vi "real time object finder single cam 2 way v2.0 EJA 09 16 2016.vi"() -> ()   [LabVIEW 2011]
doc: "The Low-Level Grab VI acquires images continuously and displays the images in an image control using low-level acquisition VIs. A grab is appropriate for high-speed applications in which you need to process only one image at a time."
uses:
  <vilib>/userdefined/High Color/IMAQdx.ctl
  <vilib>/vision/driver/IMAQdx.llb/IMAQdx Buffer Number Mode.ctl
  <vilib>/Utility/file.llb/Write To Spreadsheet File (DBL).vi
  <vilib>/vision/driver/NI_Vision_Acquisition_Software.lvlib
  resource/objmgr/imaqdx.rc
  <vilib>/Analysis/NI_AALBase.lvlib
panel:
  in  "fish size":i32=10
  out "y position histogram":T1(graph)={"X Values"=[119.25, 147.75, 176.25, 204.75, 233.25, 261.75, 290.25, 318.75, 347.25, 375.75], "Histogram: h(x)"=[6, 5, 20, 28, 28, 24, 17, 8, 6, 9]}
  out "x position histogram":T1(graph)={"X Values"=[216.3, 244.9, 273.5, 302.1, 330.7, 359.3, 387.9, 416.5, 445.1, 473.7], "Histogram: h(x)"=[6, 14, 15, 13, 13, 22, 14, 24, 18, 12]}
  in  "histogram \nbins":i32=10
  in  "always save\non stop\nimaging":bool=TRUE
  in  "acquisition \ntime (s)":i32=5
  in  "save for a \ndesignated \nperiod":bool=TRUE
  out "trajectory":cluster{i32[], i32[]}(graph)={[360, 361, 361, 360, 360, 360, 354, 347, 332, 315, 297, 296, 303, 311, 322, 333, 345, 363, 373, 383, 390, 392, 393, 394, 394, 396, 402, 407, 408, 409, 411, 397, 379, 354, 331, 304, 283, 266, 249, 233, 219, 207, 202, 204, 213, 221, 238, 265, 294, 338, 340, 352, 353, 354, 355, 356, 360, 369, 391, 412, 414, 428, 442, 446, 459, 477, 481, 484, 488, 482, 475, 469, 467, 472, 475, 470, 463, 450, 441, 428, 417, 419, 426, 427, 424, 418, 404, 383, 359, 329, 306, 287, 274, 267, 259, 259, 257, 260, 270, 287, 300, 325, 336, 334, 332, 320, 306, 299, 291, 282, 274, 269, 264, 252, 252, 252, 249, 257, 253, 245, 249, 261, 277, 296, 322, 348, 369, 391, 410, 420, 421, 421, 421, 423, 428, 431, 435, 439, 446, 454, 459, 457, 454, 451, 449, 451, 445, 437, 424, 411, 395], [247, 247, 247, 250, 252, 257, 264, 274, 280, 284, 281, 275, 265, 247, 229, 211, 204, 198, 193, 192, 192, 192, 187, 173, 154, 140, 129, 109, 105, 108, 118, 129, 140, 152, 163, 173, 176, 180, 184, 190, 201, 223, 247, 271, 301, 324, 336, 335, 328, 315, 288, 270, 255, 255, 264, 274, 284, 288, 285, 265, 250, 239, 218, 206, 215, 214, 209, 211, 202, 192, 182, 179, 182, 199, 221, 250, 268, 270, 274, 283, 285, 290, 307, 355, 362, 353, 364, 373, 382, 387, 390, 390, 382, 368, 354, 340, 322, 308, 295, 284, 281, 278, 247, 227, 202, 178, 161, 165, 178, 197, 214, 229, 246, 254, 254, 255, 256, 245, 218, 201, 198, 199, 206, 222, 229, 230, 224, 215, 201, 189, 175, 168, 165, 170, 186, 204, 221, 232, 237, 239, 239, 237, 233, 229, 228, 242, 257, 276, 295, 308, 311]}
  in  "save\nlast\nimage":bool=TRUE
  in  "stop no save":bool
  out "date stub assigned":string="_2016Y_09M_15D_09h_48m_23s"
  in  "Acquire\ndata":bool
  in  "Experimental stub":string="danio01_test"
  out "Saving":bool
  in  "save data":bool
  in  "save path":path=path "E:/danio_tracking_2016/danio01_09_14_2016"
  in  "number\nformat (%.6f)":string="%.6f"
  in  "Marker\nText color":u32(colorbox)=16711680
  out "Multiplot":cluster{cluster{dbl, i32}[]}[](graph)=[{[{0.0, 360}, {0.033, 361}, {0.066, 361}, {0.1, 360}, {0.133, 360}, {0.166, 360}, {0.199, 354}, {0.233, 347}, {0.267, 332}, {0.3, 315}, {0.333, 297}, {0.366, 296}, {0.399, 303}, {0.433, 311}, {0.466, 322}, {0.499, 333}, {0.533, 345}, {0.566, 363}, {0.6, 373}, {0.633, 383}, {0.666, 390}, {0.7, 392}, {0.733, 393}, {0.767, 394}, {0.8, 394}, {0.833, 396}, {0.866, 402}, {0.899, 407}, {0.933, 408}, {0.967, 409}, {1.0, 411}, {1.033, 397}, {1.066, 379}, {1.1, 354}, {1.133, 331}, {1.166, 304}, {1.199, 283}, {1.232, 266}, {1.267, 249}, {1.3, 233}, {1.333, 219}, {1.366, 207}, {1.399, 202}, {1.433, 204}, {1.466, 213}, {1.499, 221}, {1.532, 238}, {1.566, 265}, {1.6, 294}, {1.633, 338}, {1.666, 340}, {1.699, 352}, {1.733, 353}, {1.767, 354}, {1.8, 355}, {1.833, 356}, {1.866, 360}, {1.899, 369}, {1.933, 391}, {1.967, 412}, {2.0, 414}, {2.033, 428}, {2.066, 442}, {2.1, 446}, {2.133, 459}, {2.167, 477}, {2.2, 481}, {2.233, 484}, {2.267, 488}, {2.3, 482}, {2.333, 475}, {2.366, 469}, {2.4, 467}, {2.434, 472}, {2.467, 475}, {2.5, 470}, {2.533, 463}, {2.566, 450}, {2.6, 441}, {2.634, 428}, {2.667, 417}, {2.7, 419}, {2.733, 426}, {2.767, 427}, {2.8, 424}, {2.833, 418}, {2.866, 404}, {2.899, 383}, {2.933, 359}, {2.967, 329}, {3.0, 306}, {3.033, 287}, {3.066, 274}, {3.1, 267}, {3.133, 259}, {3.166, 259}, {3.199, 257}, {3.232, 260}, {3.266, 270}, {3.3, 287}, {3.333, 300}, {3.366, 325}, {3.399, 336}, {3.433, 334}, {3.466, 332}, {3.5, 320}, {3.533, 306}, {3.566, 299}, {3.6, 291}, {3.633, 282}, {3.666, 274}, {3.699, 269}, {3.732, 264}, {3.766, 252}, {3.8, 252}, {3.833, 252}, {3.866, 249}, {3.899, 257}, {3.933, 253}, {3.966, 245}, {3.999, 249}, {4.033, 261}, {4.066, 277}, {4.1, 296}, {4.133, 322}, {4.166, 348}, {4.2, 369}, {4.233, 391}, {4.267, 410}, {4.3, 420}, {4.333, 421}, {4.366, 421}, {4.4, 421}, {4.434, 423}, {4.467, 428}, {4.5, 431}, {4.534, 435}, {4.566, 439}, {4.6, 446}, {4.634, 454}, {4.667, 459}, {4.7, 457}, {4.733, 454}, {4.777, 451}, {4.8, 449}, {4.835, 451}, {4.867, 445}, {4.9, 437}, {4.934, 424}, {4.967, 411}, {5.0, 395}]}, {[{0.0, 247}, {0.033, 247}, {0.066, 247}, {0.1, 250}, {0.133, 252}, {0.166, 257}, {0.199, 264}, {0.233, 274}, {0.267, 280}, {0.3, 284}, {0.333, 281}, {0.366, 275}, {0.399, 265}, {0.433, 247}, {0.466, 229}, {0.499, 211}, {0.533, 204}, {0.566, 198}, {0.6, 193}, {0.633, 192}, {0.666, 192}, {0.7, 192}, {0.733, 187}, {0.767, 173}, {0.8, 154}, {0.833, 140}, {0.866, 129}, {0.899, 109}, {0.933, 105}, {0.967, 108}, {1.0, 118}, {1.033, 129}, {1.066, 140}, {1.1, 152}, {1.133, 163}, {1.166, 173}, {1.199, 176}, {1.232, 180}, {1.267, 184}, {1.3, 190}, {1.333, 201}, {1.366, 223}, {1.399, 247}, {1.433, 271}, {1.466, 301}, {1.499, 324}, {1.532, 336}, {1.566, 335}, {1.6, 328}, {1.633, 315}, {1.666, 288}, {1.699, 270}, {1.733, 255}, {1.767, 255}, {1.8, 264}, {1.833, 274}, {1.866, 284}, {1.899, 288}, {1.933, 285}, {1.967, 265}, {2.0, 250}, {2.033, 239}, {2.066, 218}, {2.1, 206}, {2.133, 215}, {2.167, 214}, {2.2, 209}, {2.233, 211}, {2.267, 202}, {2.3, 192}, {2.333, 182}, {2.366, 179}, {2.4, 182}, {2.434, 199}, {2.467, 221}, {2.5, 250}, {2.533, 268}, {2.566, 270}, {2.6, 274}, {2.634, 283}, {2.667, 285}, {2.7, 290}, {2.733, 307}, {2.767, 355}, {2.8, 362}, {2.833, 353}, {2.866, 364}, {2.899, 373}, {2.933, 382}, {2.967, 387}, {3.0, 390}, {3.033, 390}, {3.066, 382}, {3.1, 368}, {3.133, 354}, {3.166, 340}, {3.199, 322}, {3.232, 308}, {3.266, 295}, {3.3, 284}, {3.333, 281}, {3.366, 278}, {3.399, 247}, {3.433, 227}, {3.466, 202}, {3.5, 178}, {3.533, 161}, {3.566, 165}, {3.6, 178}, {3.633, 197}, {3.666, 214}, {3.699, 229}, {3.732, 246}, {3.766, 254}, {3.8, 254}, {3.833, 255}, {3.866, 256}, {3.899, 245}, {3.933, 218}, {3.966, 201}, {3.999, 198}, {4.033, 199}, {4.066, 206}, {4.1, 222}, {4.133, 229}, {4.166, 230}, {4.2, 224}, {4.233, 215}, {4.267, 201}, {4.3, 189}, {4.333, 175}, {4.366, 168}, {4.4, 165}, {4.434, 170}, {4.467, 186}, {4.5, 204}, {4.534, 221}, {4.566, 232}, {4.6, 237}, {4.634, 239}, {4.667, 239}, {4.7, 237}, {4.733, 233}, {4.777, 229}, {4.8, 228}, {4.835, 242}, {4.867, 257}, {4.9, 276}, {4.934, 295}, {4.967, 308}, {5.0, 311}]}]
  out "FPS":i32=30
  out "time (s)":dbl[](array[numeric])=[0.0, 0.033, 0.066, 0.1, 0.133, 0.166, 0.199, 0.233, 0.267, 0.3, 0.333, 0.366, 0.399, 0.433, 0.466, 0.499, 0.533, 0.566, 0.6, 0.633, 0.666, 0.7, 0.733, 0.767, 0.8, 0.833, 0.866, 0.899, 0.933, 0.967, 1.0, 1.033, 1.066, 1.1, 1.133, 1.166, 1.199, 1.232, 1.267, 1.3, 1.333, 1.366, 1.399, 1.433, 1.466, 1.499, 1.532, 1.566, 1.6, 1.633, 1.666, 1.699, 1.733, 1.767, 1.8, 1.833, 1.866, 1.899, 1.933, 1.967, 2.0, 2.033, 2.066, 2.1, 2.133, 2.167, 2.2, 2.233, 2.267, 2.3, 2.333, 2.366, 2.4, 2.434, 2.467, 2.5, 2.533, 2.566, 2.6, 2.634, 2.667, 2.7, 2.733, 2.767, 2.8, 2.833, 2.866, 2.899, 2.933, 2.967, 3.0, 3.033, 3.066, 3.1, 3.133, 3.166, 3.199, 3.232, 3.266, 3.3, 3.333, 3.366, 3.399, 3.433, 3.466, 3.5, 3.533, 3.566, 3.6, 3.633, 3.666, 3.699, 3.732, 3.766, 3.8, 3.833, 3.866, 3.899, 3.933, 3.966, 3.999, 4.033, 4.066, 4.1, 4.133, 4.166, 4.2, 4.233, 4.267, 4.3, 4.333, 4.366, 4.4, 4.434, 4.467, 4.5, 4.534, 4.566, 4.6, 4.634, 4.667, 4.7, 4.733, 4.777, 4.8, 4.835, 4.867, 4.9, 4.934, 4.967, 5.0] format="%.3f"
  in  "Origin":cluster{"X":i32, "Y":i32}
  out "Y position vs time":cluster{dbl[], i32[]}(graph)={[0.0, 0.033, 0.066, 0.1, 0.133, 0.166, 0.199, 0.233, 0.267, 0.3, 0.333, 0.366, 0.399, 0.433, 0.466, 0.499, 0.533, 0.566, 0.6, 0.633, 0.666, 0.7, 0.733, 0.767, 0.8, 0.833, 0.866, 0.899, 0.933, 0.967, 1.0, 1.033, 1.066, 1.1, 1.133, 1.166, 1.199, 1.232, 1.267, 1.3, 1.333, 1.366, 1.399, 1.433, 1.466, 1.499, 1.532, 1.566, 1.6, 1.633, 1.666, 1.699, 1.733, 1.767, 1.8, 1.833, 1.866, 1.899, 1.933, 1.967, 2.0, 2.033, 2.066, 2.1, 2.133, 2.167, 2.2, 2.233, 2.267, 2.3, 2.333, 2.366, 2.4, 2.434, 2.467, 2.5, 2.533, 2.566, 2.6, 2.634, 2.667, 2.7, 2.733, 2.767, 2.8, 2.833, 2.866, 2.899, 2.933, 2.967, 3.0, 3.033, 3.066, 3.1, 3.133, 3.166, 3.199, 3.232, 3.266, 3.3, 3.333, 3.366, 3.399, 3.433, 3.466, 3.5, 3.533, 3.566, 3.6, 3.633, 3.666, 3.699, 3.732, 3.766, 3.8, 3.833, 3.866, 3.899, 3.933, 3.966, 3.999, 4.033, 4.066, 4.1, 4.133, 4.166, 4.2, 4.233, 4.267, 4.3, 4.333, 4.366, 4.4, 4.434, 4.467, 4.5, 4.534, 4.566, 4.6, 4.634, 4.667, 4.7, 4.733, 4.777, 4.8, 4.835, 4.867, 4.9, 4.934, 4.967, 5.0], [247, 247, 247, 250, 252, 257, 264, 274, 280, 284, 281, 275, 265, 247, 229, 211, 204, 198, 193, 192, 192, 192, 187, 173, 154, 140, 129, 109, 105, 108, 118, 129, 140, 152, 163, 173, 176, 180, 184, 190, 201, 223, 247, 271, 301, 324, 336, 335, 328, 315, 288, 270, 255, 255, 264, 274, 284, 288, 285, 265, 250, 239, 218, 206, 215, 214, 209, 211, 202, 192, 182, 179, 182, 199, 221, 250, 268, 270, 274, 283, 285, 290, 307, 355, 362, 353, 364, 373, 382, 387, 390, 390, 382, 368, 354, 340, 322, 308, 295, 284, 281, 278, 247, 227, 202, 178, 161, 165, 178, 197, 214, 229, 246, 254, 254, 255, 256, 245, 218, 201, 198, 199, 206, 222, 229, 230, 224, 215, 201, 189, 175, 168, 165, 170, 186, 204, 221, 232, 237, 239, 239, 237, 233, 229, 228, 242, 257, 276, 295, 308, 311]}
  out "X position vs time":cluster{dbl[], i32[]}(graph)={[0.0, 0.033, 0.066, 0.1, 0.133, 0.166, 0.199, 0.233, 0.267, 0.3, 0.333, 0.366, 0.399, 0.433, 0.466, 0.499, 0.533, 0.566, 0.6, 0.633, 0.666, 0.7, 0.733, 0.767, 0.8, 0.833, 0.866, 0.899, 0.933, 0.967, 1.0, 1.033, 1.066, 1.1, 1.133, 1.166, 1.199, 1.232, 1.267, 1.3, 1.333, 1.366, 1.399, 1.433, 1.466, 1.499, 1.532, 1.566, 1.6, 1.633, 1.666, 1.699, 1.733, 1.767, 1.8, 1.833, 1.866, 1.899, 1.933, 1.967, 2.0, 2.033, 2.066, 2.1, 2.133, 2.167, 2.2, 2.233, 2.267, 2.3, 2.333, 2.366, 2.4, 2.434, 2.467, 2.5, 2.533, 2.566, 2.6, 2.634, 2.667, 2.7, 2.733, 2.767, 2.8, 2.833, 2.866, 2.899, 2.933, 2.967, 3.0, 3.033, 3.066, 3.1, 3.133, 3.166, 3.199, 3.232, 3.266, 3.3, 3.333, 3.366, 3.399, 3.433, 3.466, 3.5, 3.533, 3.566, 3.6, 3.633, 3.666, 3.699, 3.732, 3.766, 3.8, 3.833, 3.866, 3.899, 3.933, 3.966, 3.999, 4.033, 4.066, 4.1, 4.133, 4.166, 4.2, 4.233, 4.267, 4.3, 4.333, 4.366, 4.4, 4.434, 4.467, 4.5, 4.534, 4.566, 4.6, 4.634, 4.667, 4.7, 4.733, 4.777, 4.8, 4.835, 4.867, 4.9, 4.934, 4.967, 5.0], [360, 361, 361, 360, 360, 360, 354, 347, 332, 315, 297, 296, 303, 311, 322, 333, 345, 363, 373, 383, 390, 392, 393, 394, 394, 396, 402, 407, 408, 409, 411, 397, 379, 354, 331, 304, 283, 266, 249, 233, 219, 207, 202, 204, 213, 221, 238, 265, 294, 338, 340, 352, 353, 354, 355, 356, 360, 369, 391, 412, 414, 428, 442, 446, 459, 477, 481, 484, 488, 482, 475, 469, 467, 472, 475, 470, 463, 450, 441, 428, 417, 419, 426, 427, 424, 418, 404, 383, 359, 329, 306, 287, 274, 267, 259, 259, 257, 260, 270, 287, 300, 325, 336, 334, 332, 320, 306, 299, 291, 282, 274, 269, 264, 252, 252, 252, 249, 257, 253, 245, 249, 261, 277, 296, 322, 348, 369, 391, 410, 420, 421, 421, 421, 423, 428, 431, 435, 439, 446, 454, 459, 457, 454, 451, 449, 451, 445, 437, 424, 411, 395]}
  in  "Pixel intensity\nthreshold":i32=90
  in  "Row min":i32=10
  in  "Row max":i32=470
  in  "Column min":i32=10
  in  "Column max":i32=630
  out "X positions\ncamera 1\n(image \ncoordinates)":i32[](array[numeric])=[360, 361, 361, 360, 360, 360, 354, 347, 332, 315, 297, 296, 303, 311, 322, 333, 345, 363, 373, 383, 390, 392, 393, 394, 394, 396, 402, 407, 408, 409, 411, 397, 379, 354, 331, 304, 283, 266, 249, 233, 219, 207, 202, 204, 213, 221, 238, 265, 294, 338, 340, 352, 353, 354, 355, 356, 360, 369, 391, 412, 414, 428, 442, 446, 459, 477, 481, 484, 488, 482, 475, 469, 467, 472, 475, 470, 463, 450, 441, 428, 417, 419, 426, 427, 424, 418, 404, 383, 359, 329, 306, 287, 274, 267, 259, 259, 257, 260, 270, 287, 300, 325, 336, 334, 332, 320, 306, 299, 291, 282, 274, 269, 264, 252, 252, 252, 249, 257, 253, 245, 249, 261, 277, 296, 322, 348, 369, 391, 410, 420, 421, 421, 421, 423, 428, 431, 435, 439, 446, 454, 459, 457, 454, 451, 449, 451, 445, 437, 424, 411, 395]
  out "Y positions camera 1 \n(image \ncoordinates)":i32[](array[numeric])=[247, 247, 247, 250, 252, 257, 264, 274, 280, 284, 281, 275, 265, 247, 229, 211, 204, 198, 193, 192, 192, 192, 187, 173, 154, 140, 129, 109, 105, 108, 118, 129, 140, 152, 163, 173, 176, 180, 184, 190, 201, 223, 247, 271, 301, 324, 336, 335, 328, 315, 288, 270, 255, 255, 264, 274, 284, 288, 285, 265, 250, 239, 218, 206, 215, 214, 209, 211, 202, 192, 182, 179, 182, 199, 221, 250, 268, 270, 274, 283, 285, 290, 307, 355, 362, 353, 364, 373, 382, 387, 390, 390, 382, 368, 354, 340, 322, 308, 295, 284, 281, 278, 247, 227, 202, 178, 161, 165, 178, 197, 214, 229, 246, 254, 254, 255, 256, 245, 218, 201, 198, 199, 206, 222, 229, 230, 224, 215, 201, 189, 175, 168, 165, 170, 186, 204, 221, 232, 237, 239, 239, 237, 233, 229, 228, 242, 257, 276, 295, 308, 311]
  out "LIVE":bool
  in  "stop":bool
  out "Camera backlog":i32(slide)=-1 scale=0.0..50.0
  in  "IMAQdx Device Camera":T2="cam2"
  in  "Buffers Camera 1":u32=50
  out "Image":T3(plugin-control)
  # "PROGRAM INFO\n\nThis program finds the\nfirst pixel below the \nuser threshold in\nthe user specified\nROI below"
  # "Camera search ROI"
  # "Data acquisition \nsettings"
  # "issues\n\nHow do we know if frames \nare dropped?\n\nProbably will need to save data\nin sections to an open file\n\nCould have a sliding ROI based\non previous trailing edge position\n\nCould process each data chunk\nseparately to avoid frame dropping\nissues.  I.e. if you write every 1000\npoints, then in post processing only\nprocess 1000 at a time."
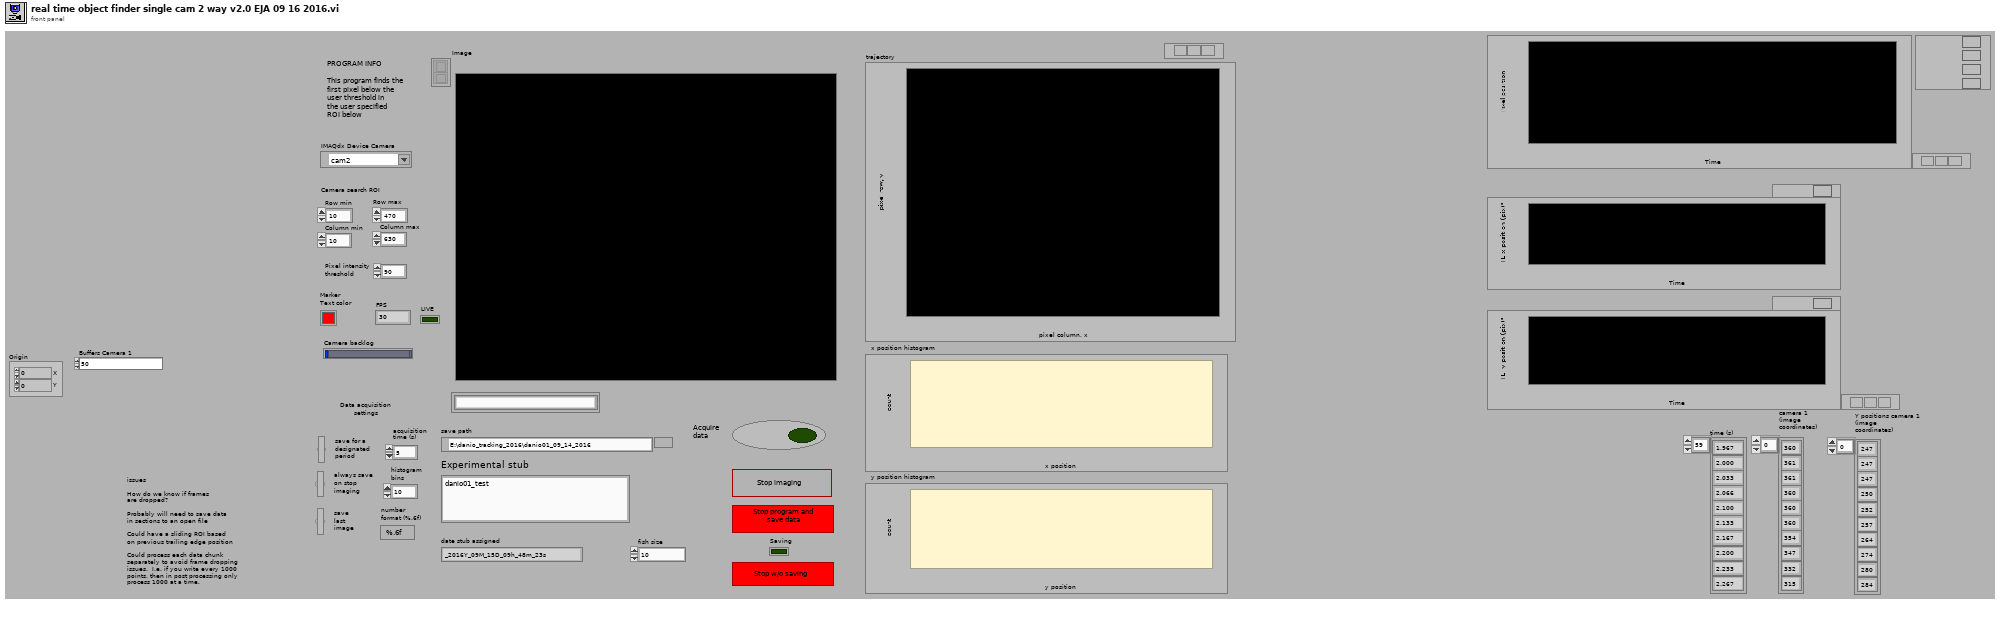
[diagram p1: front panel]
types:
  T1 = cluster{"X Values":dbl[], "Histogram: h(x)":i32[]}
  T2 = typedef "IMAQdx.ctl" = refnum<k21>
  T3 = typedef "IMAQ Image.ctl" = refnum<image>
  T4 = typedef "NI_Vision_Acquisition_Software.lvlib/IMAQdx Buffer Number Mode.ctl" = enum32{"Next", "Last", "Buffer Number"}
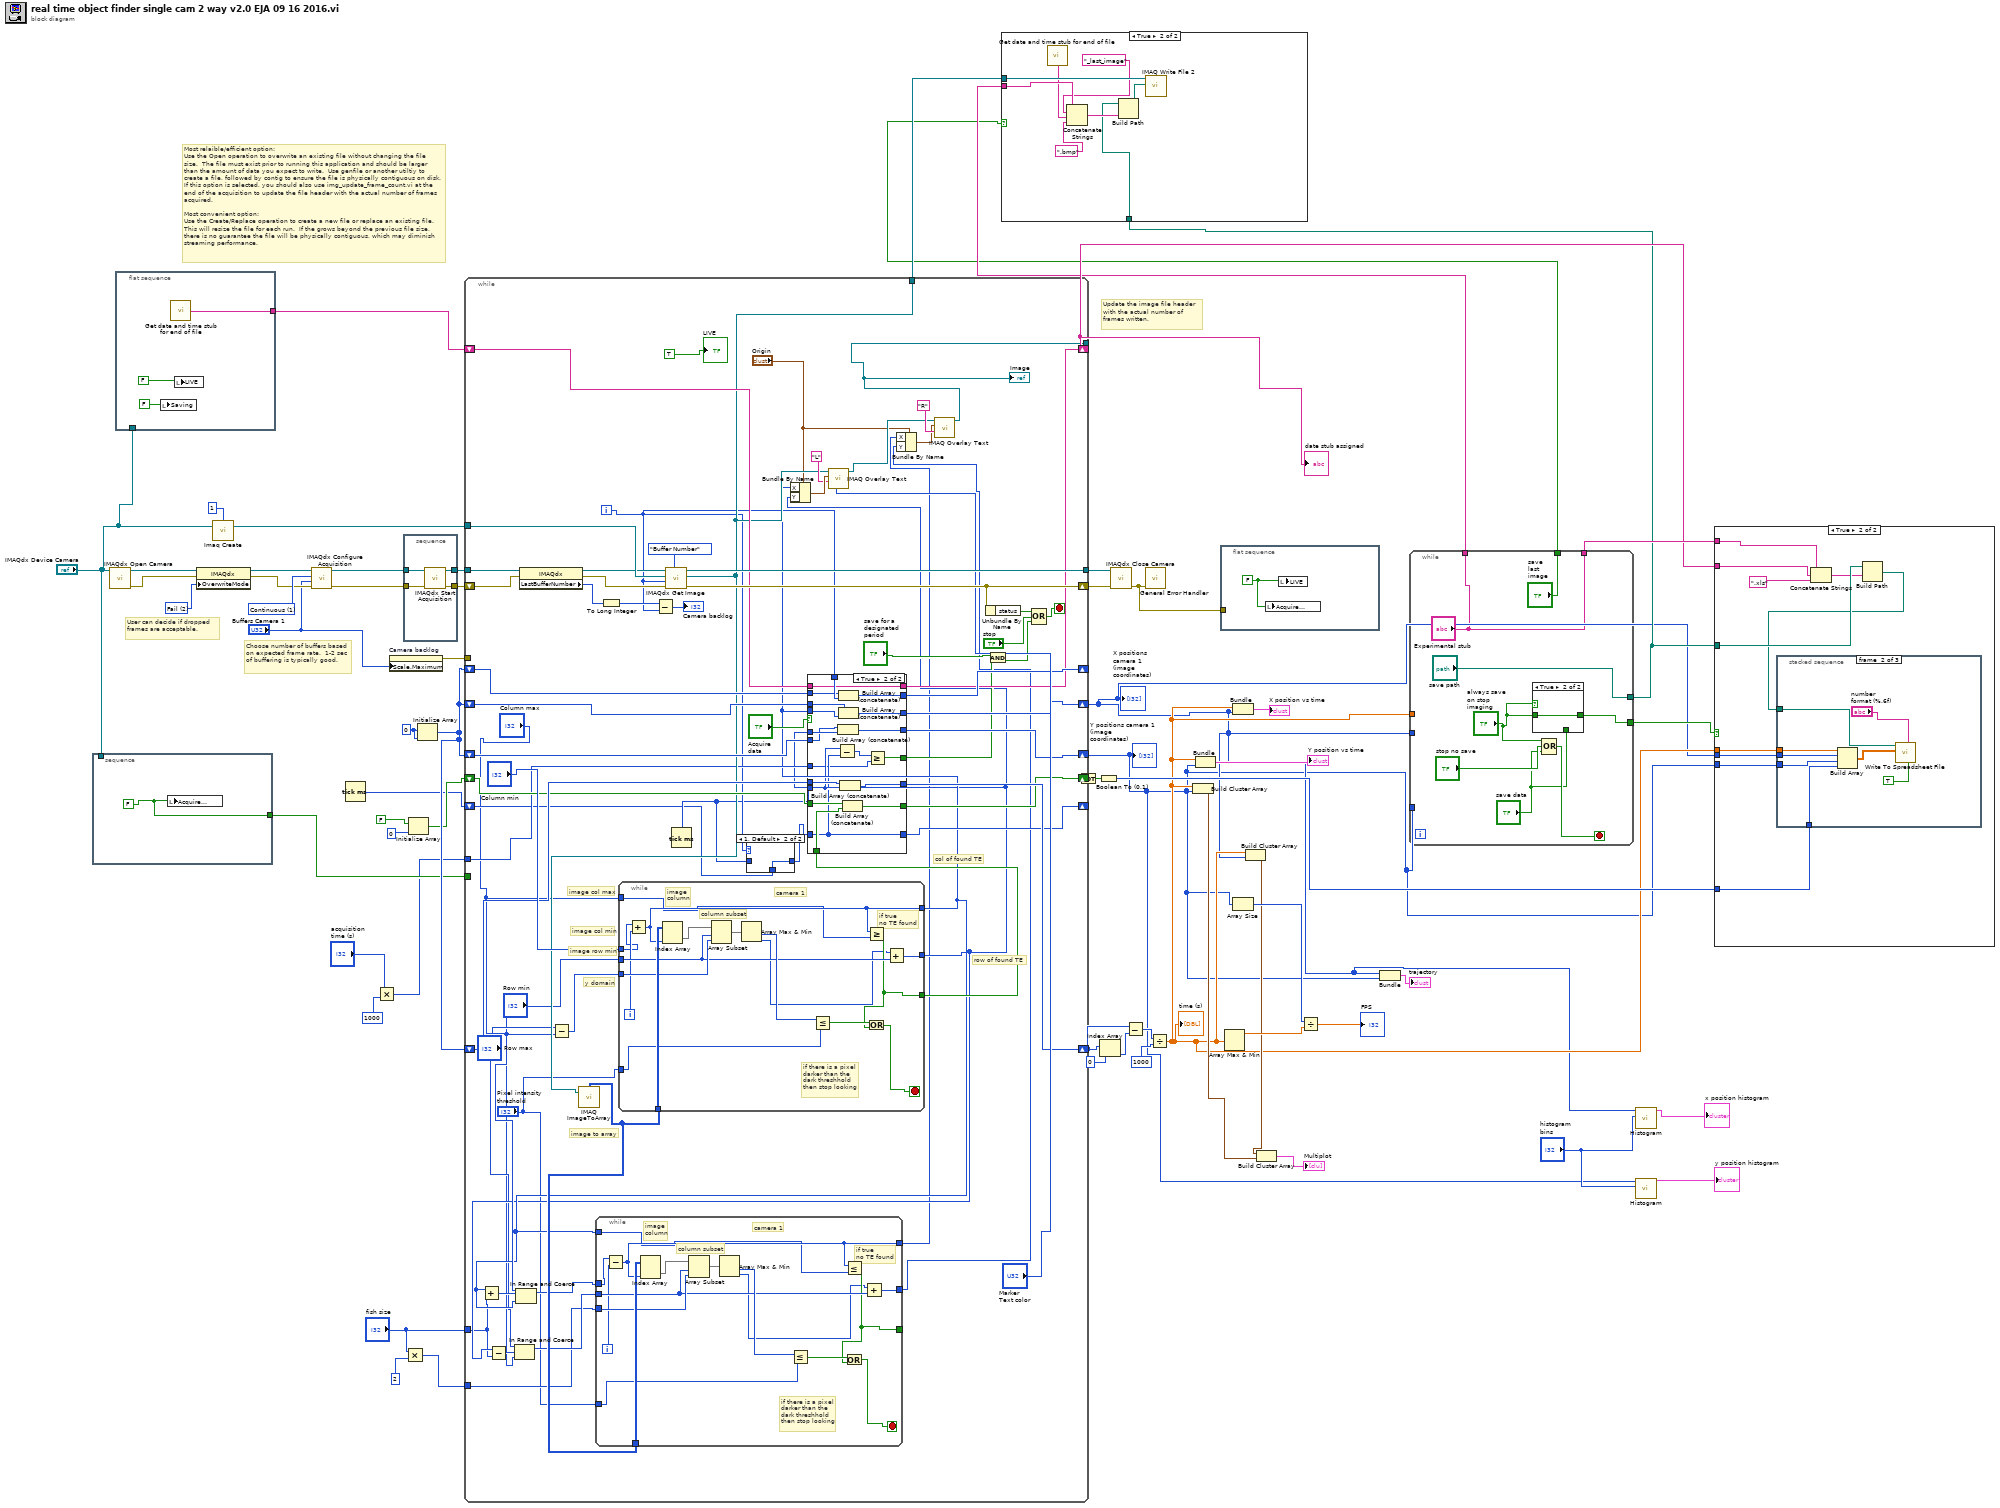
[diagram p0: block diagram]
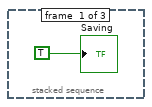
[diagram p4: hidden frame]
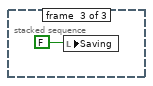
[diagram p5: hidden frame]
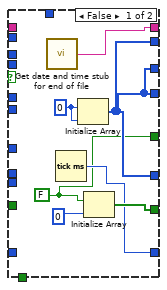
[diagram p8: hidden frame]
diagram:
  w31 = 0
  w55 = u32 2 items=["Get Oldest"=0, "Fail"=2, "Get Newest"=3] ("OverwriteMode")
  w61 = u32 1 items=["One Shot", "Continuous"] ("Continuous ?")
  # "Update the image file header with the actual number of frames written."
  # "Choose number of buffers based on expected frame rate.  1-2 sec of buffering is typically good."
  # "User can decide if dropped frames are acceptable."
  # "Most relaible/efficient option:\nUse the Open operation to overwrite an existing file without changing the file size.  The file must exist prior to running this application and should be larger than the amount of data you expect to write.  Use genfile or another utiltiy to create a file, followed by contig to ensure the file is physically contiguous on disk.  If this option is selected, you should also use img_update_frame_count.vi at the end of the acquisition to update the file header with the actual number of frames acquired. \n\nMost convenient option:\nUse the Create/Replace operation to create a new file or replace an existing file. This will resize the file for each run.  If the grows beyond the previous file size, there is no guarantee the file will be physically contiguous, which may diminish streaming performance."
  n1 = stacked-sequence {
    tunnel: "IMAQdx Device Camera" -> [_]
    tunnel: [w63] -> w15
    frame #0 {
      w63 = FALSE
      n2 = local write "Acquire\ndata"(w63) -> ()
    }
  }
  n3 = call <vilib>:"IMAQdx Open Camera.vi"("Session In"="IMAQdx Device Camera") -> ("error out"=w51:errorcluster, "Session Out"=w50:T2)  [unwired: 2 in, 7 out]
  n4 = flat-sequence {
    tunnel: "IMAQdx Device Camera" -> [_]
    tunnel: [w64] -> w30
    frame #0 {
      n5 = local write "Saving"(FALSE) -> ()
      n6 = call <userlib>:"Get date and time stub for end of file.vi"() -> ("date and time stub"=w64:string)
      n7 = local write "LIVE"(FALSE) -> ()
    }
  }
  n8 = property class="IMAQdx"(reference=w50, error in=w51, "OverwriteMode"=w55) -> (reference out=w53:T2, error out=w52:errorcluster)
  n9 = call "Imaq Create"("Border Size"=1, "Image Name"="IMAQdx Device Camera") -> ("New Image"=w62:T3)  [unwired: 2 in, 2 out]
  n10 = call <vilib>:"IMAQdx Configure Acquisition.vi"("error in"=w52, "Number of Buffers"="Buffers Camera 1", "Continuous?"=w61, "Session In"=w53) -> ("error out"=w47:errorcluster, "Session Out"=w54:T2)  [unwired: 6 out]
  n11 = Tick Count (ms)() -> (millisecond timer value=w9:u32)
  n12 = Multiply(x="acquisition \ntime (s)", y=1000) -> (x*y=w10:i32)
  n13 = property on="Camera backlog" class="Slide (strict)"("Scale.Maximum"="Buffers Camera 1") -> (error out=w49:errorcluster)  [unwired: 2 in, 1 out]
  n14 = stacked-sequence {
    tunnel: [w70] -> w60
    tunnel: [w69] -> w59
    tunnel: w54 -> [w68]
    tunnel: w47 -> [w67]
    frame #0 {
      n15 = call <vilib>:"IMAQdx Start Acquisition.vi"("error in"=w67, "Session In"=w68) -> ("error out"=w70:errorcluster, "Session Out"=w69:T2)  [unwired: 8 out]
    }
  }
  n16 = Multiply(x="fish size", y=2) -> (x*y=w1:i32)
  n17 = Initialize Array(FALSE, 0) -> (w22:bool[])
  n18 = Initialize Array(w31, w31) -> (w28:i32[])
  n19 = while {
    tunnel: [w129] -> w57
    tunnel: w59 -> [w132]
    tunnel: w62 -> [w130]
    tunnel: [w72] -> _
    shift-right: [w128] -> w56
    shift-left: w60 -> [w131]
    tunnel: w49 -> [_]
    shift-right: [w112] -> _
    shift-left: w28 -> [w113]
    shift-right: [w111] -> w8
    shift-left: w28 -> [w110]
    shift-right: [w109] -> w4
    shift-left: w28 -> [w108]
    shift-right: [w107] -> w41
    shift-left: w28 -> [w106]
    shift-right: [w104] -> w29
    shift-left: w30 -> [w105]
    shift-right: [w102] -> w27
    shift-left: w22 -> [w103]
    tunnel: [w100] -> w20
    tunnel: w15 -> [_]
    shift-right: [w99] -> _
    shift-left: w9 -> [w91]
    tunnel: w10 -> [w98]
    tunnel: "fish size" -> [w84]
    tunnel: w1 -> [w79]
    i -> [w94]
    stop <- w134 stop-if-true
    # "image col min"
    # "image col max"
    # "image row min"
    # "row of found TE"
    # "col of found TE"
    # "y domain"
    # "image to array"
    n20 = property class="IMAQdx"(reference=w132, error in=w131) -> (reference out=w125:T2, error out=w126:errorcluster, "LastBufferNumber"=w122:u32)
    n21 = Subtract(x="Row max", y="Row min") -> (x-y=w116:i32)
    n22 = To Long Integer(number=w122) -> (32bit integer=w121:i32)
    n23 = Subtract(x=w121, y=w94) -> (x-y=→"Camera backlog":i32)
    n24 = call <vilib>:"IMAQdx Get Image.vi"("Buffer Number Mode (Next)"=IMAQdx_Buffer_Number_Mode."Buffer Number", "error in"=w126, "Buffer Number In"=w94, "Image In"=w130, "Session In"=w125) -> ("error out"=w128:errorcluster, "Image Out"=w100:T3, "Session Out"=w129:T2)  [unwired: 1 in, 3 out]
    n25 = call "IMAQ ImageToArray"("Image"=w100) -> ("Image Pixels (U8)"=w90:u8[][])  [unwired: 2 in, 5 out]
    n26 = while {
      tunnel: "Row min" -> [w189]
      tunnel: [w188] -> w86
      tunnel: [w190] -> w85
      tunnel: w116 -> [w192]
      tunnel: w90 -> [w194]
      tunnel: "Column max" -> [w180]
      tunnel: "Column min" -> [w181]
      tunnel: [w185] -> w101
      tunnel: "Pixel intensity\nthreshold" -> [w183]
      i -> [w182]
      stop <- w186 stop-if-true
      # "if true\nno TE found"
      # "camera 1"
      # "if there is a pixel\ndarker than the\ndark threshhold\nthen stop looking"
      # "column subset"
      # "image\ncolumn"
      n27 = Add(x=w181, y=w182) -> (x+y=w188:i32)
      n28 = Index Array(array=w194, index (col)=w188) -> (element=w193:u8[])  [unwired: 1 in]
      n29 = Array Subset(array=w193, index=w189, length=w192) -> (w191:u8[])
      n30 = Array Max & Min(array=w191) -> (min value=w195:u8, min index (indices)=w184:i32)  [unwired: 2 out]
      n31 = Less Or Equal?(x=w195, y=w183) -> (x <= y?=w187:bool)
      n32 = Greater Or Equal?(x=w188, y=w180) -> (x >= y?=w185:bool)
      n33 = Or(x=w187, y=w185) -> (x .or. y?=w186:bool)
      n34 = Add(x=w184, y=w189) -> (x+y=w190:i32)
    }
    n35 = Add(x=w86, y=w84) -> (x+y=w89:i32)
    n36 = Subtract(x=w85, y=w84) -> (x-y=w83:i32)
    n37 = In Range and Coerce(upper limit="Row max", x=w83, lower limit="Row min") -> (coerced(x)=w80:i32)  [unwired: 1 out]
    n38 = In Range and Coerce(upper limit="Column max", x=w89, lower limit=w86) -> (coerced(x)=w87:i32)  [unwired: 1 out]
    n39 = while {
      tunnel: w80 -> [w144]
      tunnel: [w143] -> w74
      tunnel: [w145] -> w75
      tunnel: w79 -> [w147]
      tunnel: w90 -> [w149]
      tunnel: w86 -> [w135]
      tunnel: w87 -> [w136]
      tunnel: [w140] -> _
      tunnel: "Pixel intensity\nthreshold" -> [w138]
      i -> [w137]
      stop <- w141 stop-if-true
      # "if true\nno TE found"
      # "camera 1"
      # "if there is a pixel\ndarker than the\ndark threshhold\nthen stop looking"
      # "column subset"
      # "image\ncolumn"
      n40 = Subtract(x=w136, y=w137) -> (x-y=w143:i32)
      n41 = Index Array(array=w149, index (col)=w143) -> (element=w148:u8[])  [unwired: 1 in]
      n42 = Array Subset(array=w148, index=w144, length=w147) -> (w146:u8[])
      n43 = Array Max & Min(array=w146) -> (min value=w150:u8, min index (indices)=w139:i32)  [unwired: 2 out]
      n44 = Less Or Equal?(x=w150, y=w138) -> (x <= y?=w142:bool)
      n45 = Less Or Equal?(x=w143, y=w135) -> (x <= y?=w140:bool)
      n46 = Or(x=w142, y=w140) -> (x .or. y?=w141:bool)
      n47 = Add(x=w139, y=w144) -> (x+y=w145:i32)
    }
    n48 = Tick Count (ms)() -> (millisecond timer value=w93:u32)
    n49 = case shown="1, Default" w94 {
      tunnel: w93 -> [w151 _]
      tunnel: [w151 w152] -> w92
      tunnel: w91 -> [_ w152]
      frame 0 {
      }
      frame 1, Default {
      }
    }
    n50 = Bundle By Name(cluster="Origin", "X"=w86, "Y"=w85) -> (w119:cluster{"X":i32, "Y":i32})
    n51 = case shown="True" "Acquire\ndata" {
      tunnel: w94 -> [_ w179]
      tunnel: w113 -> [_ w178]
      tunnel: [w157 w177] -> w112
      tunnel: w86 -> [_ w175]
      tunnel: [w157 w176] -> w111
      tunnel: w110 -> [_ w174]
      tunnel: w85 -> [_ w173]
      tunnel: [w157 w172] -> w109
      tunnel: w108 -> [_ w171]
      tunnel: w93 -> [_ w163]
      tunnel: [w157 w170] -> w107
      tunnel: w106 -> [_ w169]
      tunnel: [w158 w168] -> w104
      tunnel: w105 -> [_ w168]
      tunnel: w103 -> [_ w167]
      tunnel: w101 -> [_ w166]
      tunnel: [w155 w165] -> w102
      tunnel: w92 -> [_ w162]
      tunnel: [w154 w162] -> w99
      tunnel: w98 -> [_ w161]
      tunnel: [w153 w160] -> w97
      frame False {
        w153 = FALSE
        w159 = 0
        n52 = call <userlib>:"Get date and time stub for end of file.vi"() -> ("date and time stub"=w158:string)
        n53 = Tick Count (ms)() -> (millisecond timer value=w154:u32)
        n54 = Initialize Array(w159, w159) -> (w157:i32[])
        n55 = Initialize Array(w153, 0) -> (w155:bool[])
      }
      frame True {
        n56 = Subtract(x=w163, y=w162) -> (x-y=w164:u32)
        n57 = Build Array (concatenate)(w171, w173) -> (w172:i32[])
        n58 = Build Array (concatenate)(w178, w179) -> (w177:i32[])
        n59 = Build Array (concatenate)(w174, w175) -> (w176:i32[])
        n60 = Build Array (concatenate)(w169, w163) -> (w170:u32[])
        n61 = Build Array (concatenate)(w167, w166) -> (w165:bool[])
        n62 = Greater Or Equal?(x=w164, y=w161) -> (x >= y?=w160:bool)
      }
    }
    n63 = call "IMAQ Overlay Text"("Text Color (black)"="Marker\nText color", "String"="L", "Origin"=w119, "Image"=w100) -> ("Image Out"=w73:T3)  [unwired: 4 in, 3 out]
    n64 = Bundle By Name(cluster="Origin", "X"=w74, "Y"=w75) -> (w76:cluster{"X":i32, "Y":i32})
    n65 = call "IMAQ Overlay Text"("String"="R", "Origin"=w76, "Image"=w73) -> ("Image Out"=w72:T3)  [unwired: 5 in, 3 out]
    "Image" <- w72
    n66 = Unbundle By Name(w128) -> ("status"=w133:bool)
    n67 = And(x="save for a \ndesignated \nperiod", y=w97) -> (x .and. y?=w96:bool)
    n68 = Compound Arithmetic op=OR(w133, "stop", w96) -> (w134:bool)
    "LIVE" <- TRUE
  }
  "X positions\ncamera 1\n(image \ncoordinates)" <- w8
  "Y positions camera 1 \n(image \ncoordinates)" <- w4
  "date stub assigned" <- w29
  n69 = Not(x=w27) -> (.not. x?=w24:bool[])
  n70 = Boolean To (0,1)(Boolean=w24) -> (0, 1=w23:i16[])
  n71 = Index Array(array=w41, index=0) -> (element=w42:u32)
  n72 = call <vilib>:"IMAQdx Close Camera.vi"("error in"=w56, "Session In"=w57) -> ("error out"=w46:errorcluster)  [unwired: 9 out]
  n73 = Subtract(x=w41, y=w42) -> (x-y=w36:u32[])
  n74 = call <vilib>:"General Error Handler.vi"("error in (no error)"=w46) -> ()  [unwired: 1 in, 14 out]
  n75 = Divide(x=w36, y=1000) -> (x/y=w14:dbl[])
  "time (s)" <- w14
  n76 = Build Cluster Array(w14, w4) -> (w33:cluster{dbl, i32}[])
  n77 = Bundle(w14, w4) -> (→"Y position vs time":cluster{dbl[], i32[]})  [unwired: 1 out]
  n78 = flat-sequence {
    tunnel: w46 -> [_]
    frame #0 {
      w196 = FALSE
      n79 = local write "Acquire\ndata"(w196) -> ()
      n80 = local write "LIVE"(w196) -> ()
    }
  }
  n81 = Array Max & Min(array=w14) -> (max value=w40:dbl)  [unwired: 3 out]
  n82 = Bundle(w14, w8) -> (→"X position vs time":cluster{dbl[], i32[]})  [unwired: 1 out]
  n83 = Array Size(array=w4) -> (size(s)=w39:i32)
  n84 = Build Cluster Array(w14, w8) -> (w34:cluster{dbl, i32}[])
  n85 = Build Cluster Array(w34, w33) -> (→"Multiplot":cluster{cluster{dbl, i32}[]}[])
  n86 = Divide(x=w39, y=w40) -> (x/y=→"FPS":dbl)
  n87 = Bundle(w8, w4) -> (→"trajectory":cluster{i32[], i32[]})  [unwired: 1 out]
  n88 = while {
    tunnel: w14 -> [_]
    tunnel: w8 -> [_]
    tunnel: w4 -> [_]
    tunnel: ["save path"] -> w18
    tunnel: ["Experimental stub"] -> w32
    tunnel: [w198] -> w21
    tunnel: ["Experimental stub"] -> w19
    tunnel: ["save\nlast\nimage"] -> w17
    stop <- w200 stop-if-true
    n89 = case shown="True" "always save\non stop\nimaging" {
      tunnel: [w205 w206] -> w198
      tunnel: "always save\non stop\nimaging" -> [_ w206]
      tunnel: "save data" -> [w205 _]
      frame False {
      }
      frame True {
      }
    }
    n90 = Compound Arithmetic op=OR("always save\non stop\nimaging", "stop no save", "save data") -> (w200:bool)
  }
  n91 = case shown="True" w17 {
    tunnel: w20 -> [_ w214]
    tunnel: w19 -> [_ w212]
    tunnel: w18 -> [_ w207]
    frame False {
    }
    frame True {
      n92 = call <userlib>:"Get date and time stub for end of file.vi"() -> ("date and time stub"=w210:string)
      n93 = Concatenate Strings(w212, "_last_image", w210, ".bmp") -> (w213:string)
      n94 = Build Path(base path=w207, name or relative path=w213) -> (appended path=w208:path)
      n95 = call-poly "IMAQ Write File 2"("File Path"=w208, "Image"=w214) -> ()  [unwired: 8 in, 2 out]
    }
  }
  n96 = call <vilib>:"Histogram.vi"("intervals"="histogram \nbins", "X"=w8) -> ("Histogram Graph"=→"x position histogram":T1)  [unwired: 6 in, 3 out]
  n97 = call <vilib>:"Histogram.vi"("intervals"="histogram \nbins", "X"=w4) -> ("Histogram Graph"=→"y position histogram":T1)  [unwired: 6 in, 3 out]
  n98 = case shown="True" w21 {
    tunnel: w14 -> [_ w224]
    tunnel: w8 -> [_ w223]
    tunnel: w4 -> [_ w222]
    tunnel: w32 -> [_ w220]
    tunnel: w18 -> [_ w219]
    tunnel: w29 -> [_ w216]
    tunnel: w23 -> [_ w215]
    frame False {
    }
    frame True {
      n99 = Concatenate Strings(w220, w216, ".xls") -> (w218:string)
      n100 = Build Path(base path=w219, name or relative path=w218) -> (appended path=w217:path)
      n101 = stacked-sequence {
        tunnel: w217 -> [_ w231 _]
        tunnel: w224 -> [_ w230 _]
        tunnel: w223 -> [_ w229 _]
        tunnel: w222 -> [_ w228 _]
        tunnel: w215 -> [_ w227 _]
        frame #0 {
          "Saving" <- TRUE
        }
        frame #1 {
          n102 = Build Array(w230, w229, w228, w227) -> (w226:dbl[][])
          n103 = call-poly <vilib>:"Write To Spreadsheet File.vi"("transpose? (no:F)"=TRUE, "format (%.3f)"="number\nformat (%.6f)", "2D data"=w226, "file path (dialog if empty)"=w231) -> ()  [unwired: 4 in, 1 out]
        }
        frame #2 {
          n104 = local write "Saving"(FALSE) -> ()
        }
      }
    }
  }
